vi "Pockels_FPGA.vi"(8 "error in (no error)":errorcluster, 9 "Laser(V)":dbl format="%#_13g", 10 "Pockels Mode_FPGA":T1(ring)=enum."Modulate", 11 "Imaging Protocol":T2=enum."Live Imaging") -> (0 "error out":errorcluster, 3 "Pockels Packet":string)   [LabVIEW 2017]
uses:
  Typedefs/Imaging Protocols enum.ctl
  Global Variables/General Globals.vi
panel:
  out "number":u32
  out "bin_in":bool[](array[boolean])
  out "bin_out_invert_14":bool[](array[boolean])
  out "Hex string 2":string
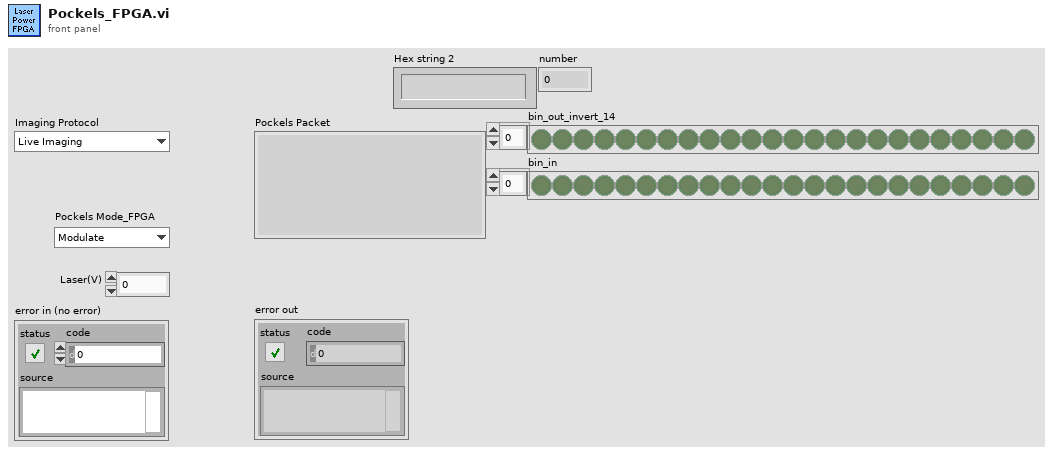
[diagram p1: front panel]
types:
  T1 = enum8{"Clear the register", "Always ON", "Modulate"}
  T2 = typedef "Imaging Protocols enum.ctl" = enum16{"AOL Z-Stack", "Motor Z Stack", "Functional Acquisition", "Single Plane Acquisition", "Volume Acquisition", "Live Imaging", "Live Plane Imaging", "Live Volume Imaging"}
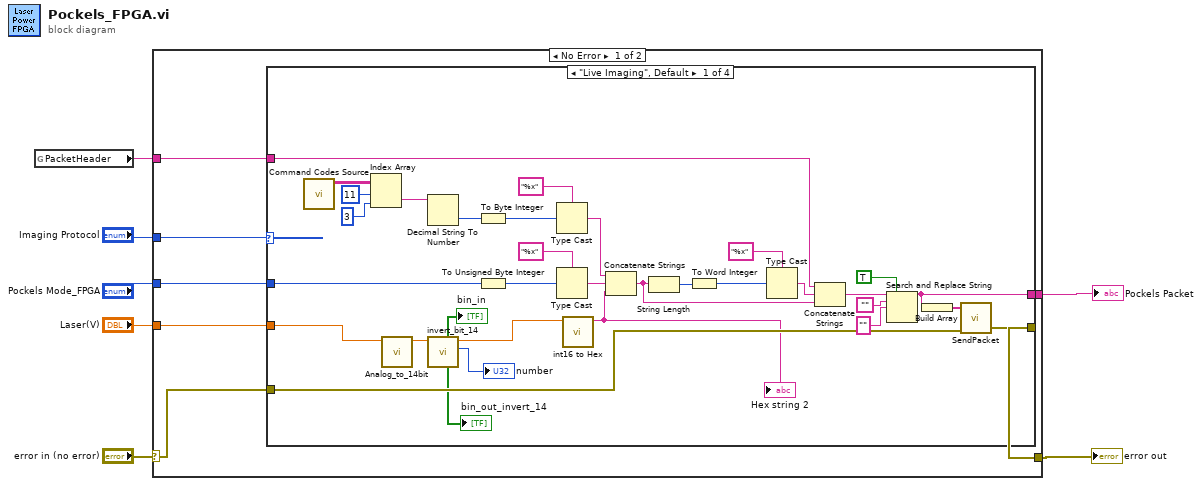
[diagram p0: block diagram]
diagram:
  n1 = global read "General Globals.vi" "PacketHeader"() -> (w2:string)
  n2 = case shown="No Error" "error in (no error)" {
    selector: "error in (no error)" -> [w8 w51]
    tunnel: "Imaging Protocol" -> [w14 _]
    tunnel: [w9 w51] -> w5
    tunnel: "Laser(V)" -> [w13 _]
    tunnel: "Pockels Mode_FPGA" -> [w12 _]
    tunnel: w2 -> [w11 _]
    tunnel: [w10 _] -> w1
    frame No Error {
      n3 = case shown="\"Live Imaging\", Default" w14 {
        tunnel: w13 -> [w20 _ _ _]
        tunnel: w12 -> [w27 _ _ _]
        tunnel: w11 -> [w26 _ _ _]
        tunnel: [w24 _ _ _] -> w10
        tunnel: [w23 w48 w49 w50] -> w9
        tunnel: w8 -> [w22 w48 w49 w50]
        frame "Live Imaging", Default {
          n4 = call "Command Codes Source.vi"() -> ("Commands for FPGA"=w36:string[][])  [unwired: 11 in]
          n5 = Index Array(array=w36, index (row)=11 ("disabled index (row)"), index (col)=3 ("disabled index (col)")) -> (element=w39:string)
          n6 = call "Analog_to_14bit.vi"("Pockels (0-2V)"=w20) -> ("Pockels Level(14 bit)"=w19:dbl)  [unwired: 10 in]
          n7 = Decimal String To Number(string=w39) -> (number=w37:i32)  [unwired: 2 in, 1 out]
          n8 = call "invert_bit_14.vi"("Pockels Level(14 bit)"=w19) -> ("number"=→"number":u32, "to hex convert"=w18:dbl, "bin_out_invert_14"=→"bin_out_invert_14":bool[], "bin_in"=→"bin_in":bool[])  [unwired: 7 in]
          n9 = To Byte Integer(number=w37) -> (8bit integer=w38:i8)
          n10 = To Unsigned Byte Integer(number=w27) -> (unsigned 8bit integer=w45:u8)
          n11 = Type Cast(type="%x", x=w38) -> (*(type *) &x=w40:string)
          n12 = Type Cast(type="%x", x=w45) -> (*(type *) &x=w46:string)
          n13 = call "int16 to Hex.vi"("number"=w18) -> ("Hex string"=w21:string)  [unwired: 10 in]
          "Hex string 2" <- w21
          n14 = Concatenate Strings(w40, w46, w21) -> (w47:string)
          n15 = String Length(string=w47) -> (length=w41:i32)
          n16 = To Word Integer(number=w41) -> (16bit integer=w42:i16)
          n17 = Type Cast(type="%x", x=w42) -> (*(type *) &x=w43:string)
          n18 = Concatenate Strings(w26, w43, w47) -> (w44:string)
          n19 = Search and Replace String(replace all?=TRUE ("replace all? (F)"), input string=w44, search string="", replace string="" ("replace string (\"\")")) -> (result string=w24:string)  [unwired: 4 in, 3 out]
          n20 = Build Array(w24) -> (w25:string[])
          n21 = call "SendPacket.vi"("error in"=w22, "Packet Array"=w25) -> ("error out"=w23:errorcluster)  [unwired: 8 in, 1 out]
        }
        frame "AOL Z-Stack" {
        }
        frame "Functional Acquisition" {
        }
        frame "Motor Z Stack" {
        }
      }
    }
    frame Error {
    }
  }
  "error out" <- w5
  "Pockels Packet" <- w1
